vi "ConfigureContinuous.vi"(8 "error in (no error)":errorcluster, 10 "on demand acq config":T4, 11 "config":T1) -> (0 "error out":errorcluster, 3 "config out":T1)   [LabVIEW 2017, in "EmsaAcquisition.lvlib"]
uses:
  <vilib>/addons/InsightCM/Devices/Shared/Emsa/EmsaAcquisition/EmsaAcquisition.lvlib
  <vilib>/addons/InsightCM/Devices/Shared/Emsa/EmsaAcquisition/controls/StartOnDemandAcquisitionRoutedMessage.ctl
  <vilib>/addons/InsightCM/Devices/Shared/Emsa/EmsaAcquisition/controls/config.ctl
  <vilib>/addons/InsightCM/Devices/Shared/Emsa/Emsa9770API/9770 API.lvclass
  <vilib>/addons/InsightCM/Devices/Shared/Emsa/EmsaAcquisition/controls/group.ctl
  <vilib>/addons/InsightCM/Devices/Shared/Emsa/EmsaAcquisition/controls/acqConfig.ctl
  <vilib>/LabVIEW Targets/FPGA/cRIO/shared/nicrio_ModuleControls/nicrio_cRIO-9770_DataRatesRing.ctl
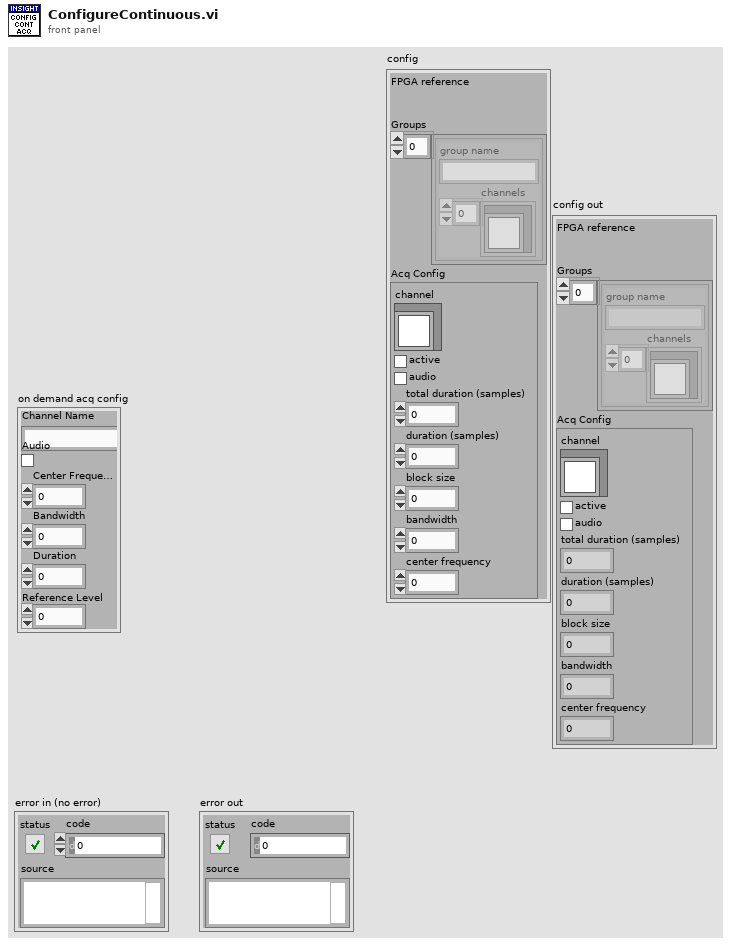
[diagram p1: front panel]
types:
  T1 = typedef "EmsaAcquisition.lvlib/config.ctl" = cluster{"FPGA reference":refnum<k20>, "Groups":T2[], "Acq Config":T3}
  T2 = typedef "EmsaAcquisition.lvlib/group.ctl" = cluster{"group name":string, "channels":refnum<class "9770 API.lvclass">[]}
  T3 = typedef "EmsaAcquisition.lvlib/acqConfig.ctl" = cluster{"channel":refnum<class "9770 API.lvclass">, "active":bool, "audio":bool, "total duration (samples)":i32, "duration (samples)":i32, "block size":i32, "bandwidth":dbl, "center frequency":dbl}
  T4 = typedef "EmsaAcquisition.lvlib/StartOnDemandAcquisitionRoutedMessage.ctl" = cluster{"Channel Name":string, "Audio":bool, "Center Frequency":dbl, "Bandwidth":dbl, "Duration":dbl, "Reference Level":dbl}
  T5 = typedef "nicrio_cRIO-9770_DataRatesRing.ctl" = u8
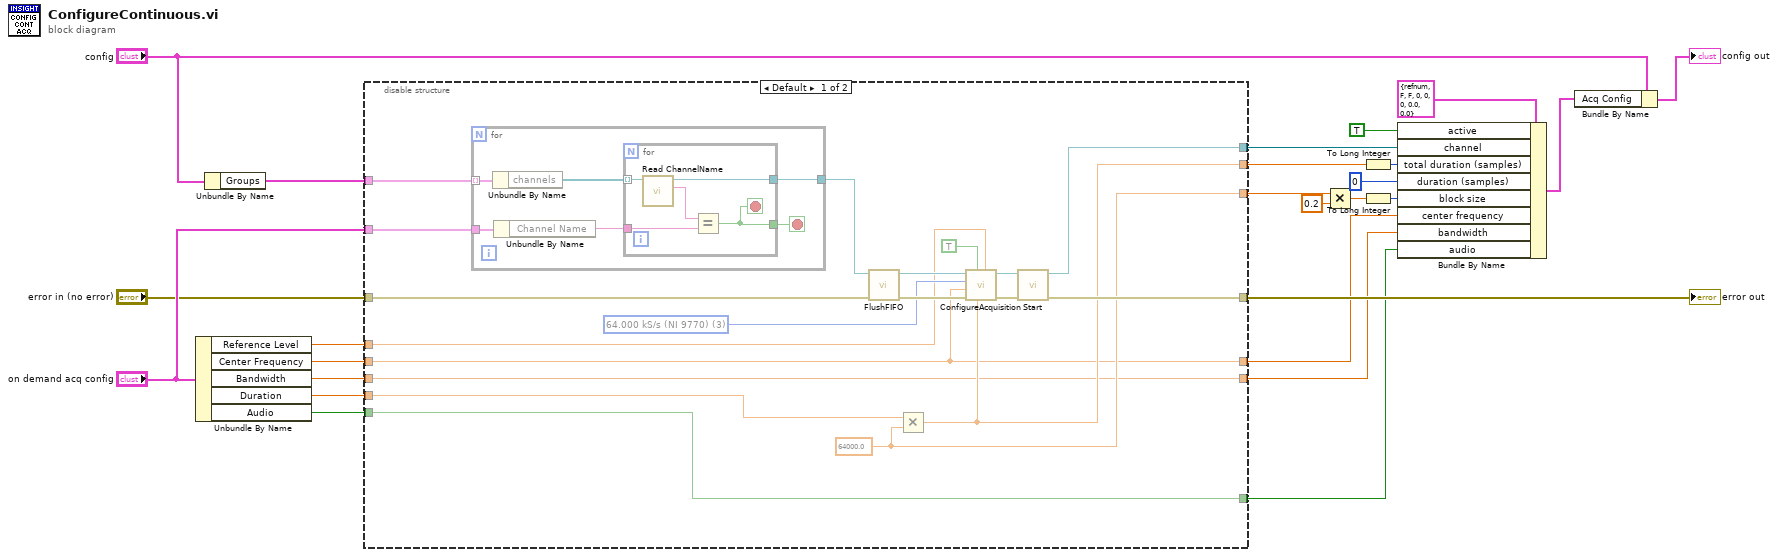
[diagram p0: block diagram]
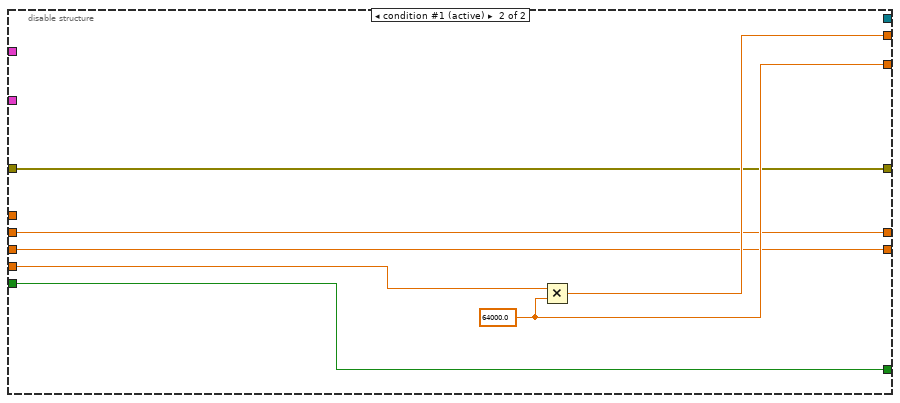
[diagram p2: hidden frame]
diagram:
  n1 = Unbundle By Name("on demand acq config") -> ("Reference Level"=w10:dbl, "Center Frequency"=w25:dbl, "Bandwidth"=w3:dbl, "Duration"=w6:dbl, "Audio"=w1:bool)
  n2 = Unbundle By Name("config") -> ("Groups"=w18:T2[])
  n3 = disable-structure shown="Default" {
    disable-tunnel: w25 -> [w28 w59]
    disable-tunnel: [w44 w56] -> w24
    disable-tunnel: [w38 w62] -> w22
    disable-tunnel: "on demand acq config" -> [w35 _]
    disable-tunnel: "error in (no error)" -> [w34 w56]
    disable-tunnel: w18 -> [w33 _]
    disable-tunnel: [w32 _] -> w16
    disable-tunnel: [w31 w61] -> w14
    disable-tunnel: w10 -> [w30 _]
    disable-tunnel: w6 -> [w29 w60]
    disable-tunnel: w1 -> [w26 w57]
    disable-tunnel: [w28 w59] -> w5
    disable-tunnel: [w27 w58] -> w4
    disable-tunnel: w3 -> [w27 w58]
    disable-tunnel: [w26 w57] -> w2
    frame condition #0 {
      w38 = 64000.0 ("y")
      w36 = T5 3 items=["320.000 kS/s (NI 9770)", "256.000 kS/s (NI 9770)", "128.000 kS/s (NI 9770)", "64.000 kS/s (NI 9770)", "32.000 kS/s (NI 9770)", "16.000 kS/s (NI 9770)", "8.000 kS/s (NI 9770)", "4.000 kS/s (NI 9770)"] ("Data Rate")
      n4 = for {
        tunnel: w33 -> [w50] mode=indexing
        tunnel: w35 -> [w49]
        tunnel: [w45] -> w39
        stop <- w46 stop-if-true
        n5 = Unbundle By Name(w50) -> ("channels"=w48:refnum<class "9770 API.lvclass">[])
        n6 = Unbundle By Name(w49) -> ("Channel Name"=w47:string)
        n7 = for {
          tunnel: w48 -> [w55] mode=indexing
          tunnel: w47 -> [w53]
          tunnel: [w52] -> w45
          tunnel: [w51] -> w46
          stop <- w51 stop-if-true
          n8 = call <vilib>:"Read ChannelName.vi"("9770 API in"=w55) -> ("ChannelName"=w54:string, "9770 API out"=w52:refnum<class "9770 API.lvclass">)  [unwired: 8 in, 1 out]
          n9 = Equal?(x=w54, y=w53) -> (x = y?=w51:bool)
        }
      }
      n10 = call <vilib>:"FlushFIFO.vi"("error in (no error)"=w34, "9770 API in"=w39) -> ("error out"=w40:errorcluster, "9770 API out"=w41:refnum<class "9770 API.lvclass">)  [unwired: 8 in]
      n11 = Multiply(x=w29, y=w38) -> (x*y=w31:dbl)
      n12 = call <vilib>:"ConfigureAcquisition.vi"("Reference Level (dBm)"=w30, "Number of Samples"=w31, "Continuous"=TRUE, "error in (no error)"=w40, "Center Frequency (Hz)"=w28, "Data Rate"=w36, "9770 API in"=w41) -> ("error out"=w42:errorcluster, "9770 API out"=w43:refnum<class "9770 API.lvclass">)  [unwired: 3 in]
      n13 = call-dynamic "Start.vi"("error in (no error)"=w42, "RIO_API in"=w43) -> ("error out"=w44:errorcluster, "RIO_API out"=w32:refnum<class "9770 API.lvclass">)  [unwired: 8 in]
    }
    frame condition #1 (active) {
      w62 = 64000.0 ("y")
      n14 = Multiply(x=w60, y=w62) -> (x*y=w61:dbl)
    }
  }
  "error out" <- w24
  n15 = Multiply(x=w22, y=0.2) -> (x*y=w12:dbl)
  n16 = To Long Integer(number=w14) -> (32bit integer=w13:i32)
  n17 = To Long Integer(number=w12) -> (32bit integer=w11:i32)
  n18 = Bundle By Name(cluster=T3 {"channel"=refnum, "active"=FALSE, "audio"=FALSE, "total duration (samples)"=0, "duration (samples)"=0, "block size"=0, "bandwidth"=0.0, "center frequency"=0.0} ("Acq Config"), "active"=TRUE, "channel"=w16, "total duration (samples)"=w13, "duration (samples)"=0, "block size"=w11, "center frequency"=w5, "bandwidth"=w4, "audio"=w2) -> (w8:T3)
  n19 = Bundle By Name(cluster="config", "Acq Config"=w8) -> (→"config out":T1)
